vi "Create Tag Path.vi"(8 "error in (no error)":errorcluster, 10 "namespace":string, 11 "tag name":string) -> (0 "error out":errorcluster, 3 "path":string)   [LabVIEW 2017, in "Logger.lvclass"]
uses:
  logger/Logger.lvclass
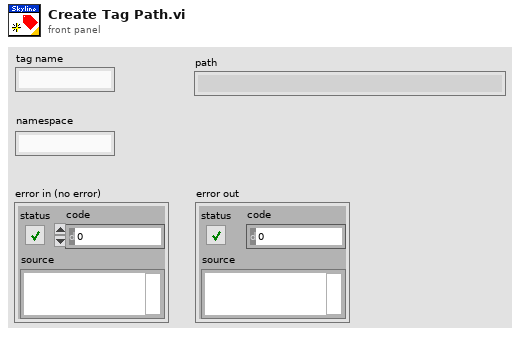
[diagram p1: front panel]
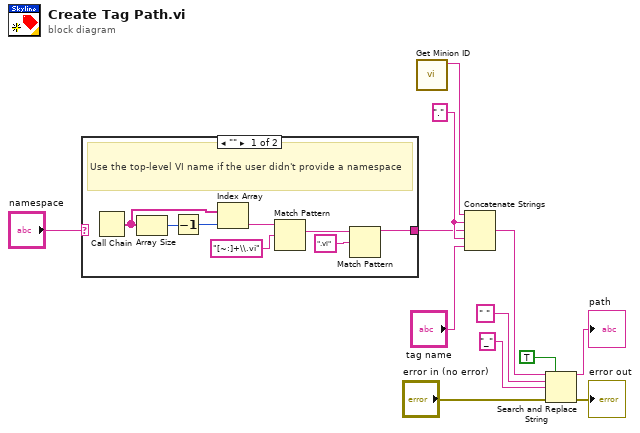
[diagram p0: block diagram]
diagram:
  w3 = "." ("element")
  n1 = case shown="\"\"" "namespace" {
    selector: "namespace" -> [_ w21]
    tunnel: [w13 w21] -> w1
    frame "" {
      # "Use the top-level VI name if the user didn't provide a namespace"
      n2 = Call Chain() -> (call chain=w16:string[])
      n3 = Array Size(array=w16) -> (size(s)=w17:i32)
      n4 = Decrement(x=w17) -> (x-1=w18:i32)
      n5 = Index Array(array=w16, index=w18) -> (element=w19:string)
      n6 = Match Pattern(string=w19, regular expression="[~:]+\\.vi") -> (match substring=w20:string)  [unwired: 1 in, 3 out]
      n7 = Match Pattern(string=w20, regular expression=".vi") -> (before substring=w13:string)  [unwired: 1 in, 3 out]
    }
    frame "valid", Default {
    }
  }
  n8 = call "Get Minion ID.vi"() -> ("minion id"=w2:string)  [unwired: 11 in]
  n9 = Concatenate Strings(w2, w3, w1, w3, "tag name") -> (w4:string)
  n10 = Search and Replace String(replace all?=TRUE ("replace all? (F)"), input string=w4, search string=" ", replace string="_" ("replace string (\"\")"), error in="error in (no error)") -> (result string=→"path":string, error out=→"error out":errorcluster)  [unwired: 3 in, 2 out]
